vi "Channel Global.vi"() -> ()   [LabVIEW 2016, in "Control Experiment.lvclass"]
uses:
  Control Experiment.lvclass
panel:
  in  "V4-":i32=1
  in  "V4+":i32
  in  "Vsg1":i32=1
  in  "V3-":i32=2
  in  "V3+":i32=1
  in  "V2-":i32=3
  in  "V2+":i32=2
  in  "V1-":i32=1
  in  "V1+":i32=2
  in  "I-":i32=6
  in  "I+":i32=2
  # "PPMS2 \nDevice Configuration\nChannel number running from 0 to 7, corresponding to KH 1 to 8."
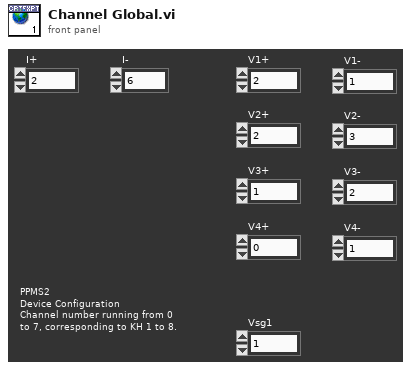
[diagram p1: front panel]
diagram:
